vi "Perform actrion and wait for responce.vi"(7 "data step cluster":T1, 11 "error in (no error)":errorcluster) -> (2 "Rdesistance go to":bool, 3 "Voltage go to":bool, 6 "Continue":bool, 8 "Retry":bool, 13 "Stroke  go to":bool, 14 "Action value tool":dbl, 15 "error out":errorcluster)   [LabVIEW 2011]
uses:
  Sequence steps config..ctl
  Single criteria cluster.ctl
  Criteria types.ctl
  Boolean operation.ctl
  Measurments Handling/Action Analog Handler.ctl
  Measurments Handling/Common/Variable List Common Digital.ctl
  Measurments Handling/Status Digitalish.ctl
  Tool/Stroker/def/Tool specific commands.ctl
  PCP interface/High Level/PCP High Level Commands.ctl
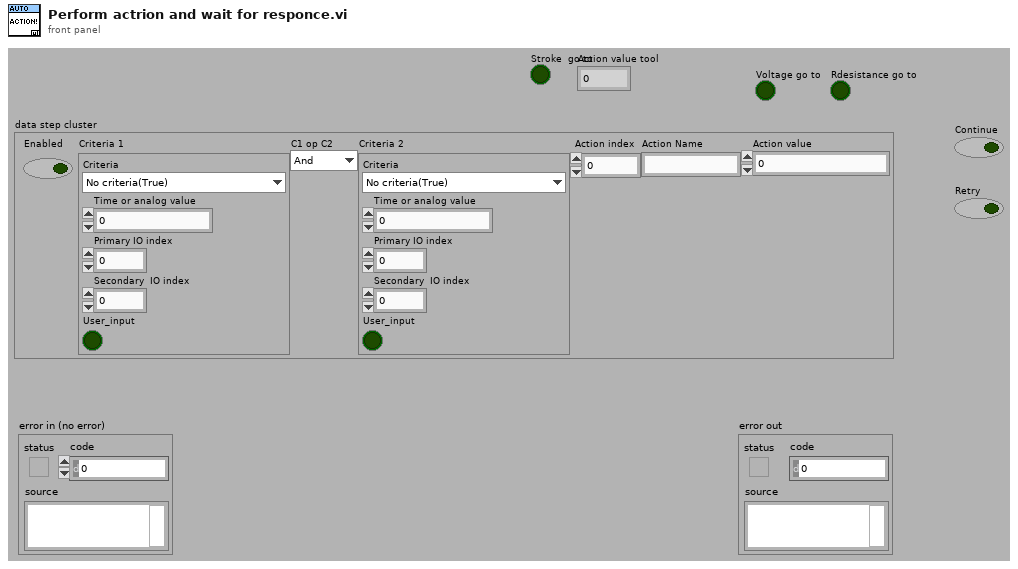
[diagram p1: front panel]
types:
  T1 = typedef "Sequence steps config..ctl" = cluster{"Enabled":bool, "Criteria 1":T2, "C1 op C2":T4, "Criteria 2":T2, "Action index":i32, "Action Name":string, "Action value":dbl}
  T2 = typedef "Single criteria cluster.ctl" = cluster{"Criteria":T3, "Time or analog value":dbl, "Primary IO index":i32, "Secondary  IO index":i32, "User_input":bool}
  T3 = typedef "Criteria types.ctl" = enum16{"No criteria(True)", "Time(s)", "Analog IO over", "Analog IO over or equal", "Analog IO under", "Analog IO under or equal", "Analog IO 1 minus Analog IO 2 over", "Digital IO True", "Digital IO False", "Operator approval"}
  T4 = typedef "Boolean operation.ctl" = enum16{"And", "Or", "Xor", "Nand", "Nor", "Nxor", "Implies"}
  T5 = typedef "PCP High Level Commands.ctl" = enum16{"HVPSU HV ON", "HVPSU HV OFF", "PCP PC", "PCP Local", "Update Motor Voltage", "Update Cable Resistance", "Final Motor Voltage", "Final Resistance"}
  T6 = typedef "Tool specific commands.ctl" = enum16{"controller relay 1 on", "controller relay 1 off", "controller relay 2 on", "controller relay 2 off", "Solonoid 1 (master) on", "Solonoid 1 (master) off", "Solonoid 2 (Stroker) on", "Solonoid 2 (Stroker) off", "Solonoid 3 (Anchor) on", "Solonoid 3 (Anchor) off", "Controller relay 1 & 2 on", "Controller relay 1 & 2 off", "Controller relay 1 on, 2 off", "Controller relay 1 off, 2 on", "STROKER tool: Stop Force Mon", "High-G Stop", "High-G Get data", "High-G Stop Get data", "STROKER tool: Stroke out", "STROKER tool: Stroke in", "STROKER tool: Stroke stop", "STROKER tool: Stroke go to", "STROKER tool: Stop Homing", "STROKER tool: Start Force Mon dir in", "STROKER tool: Start Force Mon dir out", "Controller STOP"}
  T7 = typedef "Status Digitalish.ctl" = enum16{"NA", "False", "True"}
  T8 = typedef "Variable List Common Digital.ctl" = enum16{"PCP Connected", "PCP PC Control", "HV PSU connected", "HV PSU HV Active", "Modem Connected", "Tool Connected", "CanBus interface"}
  T9 = typedef "Action Analog Handler.ctl" = enum16{"GET value", "GET Single Frequenzy", "GET All Values", "GET Waveform", "Get Numb Var", "SET Value", "START Buffer", "REG Variable", "BUF size(total antal sekund)", "PULS", "Get a Value at time", "Set initial waveform"}
  T10 = typedef "Action colleciton cluster.ctl" = cluster{"common":T11, "Action type":T13, "General command":T14, "PCP command":T5, "Tool command":T6}
  T11 = typedef "Action common elements.ctl" = cluster{"Name":string, "Adjuster type":T12, "Adjuster double default value":dbl}
  T12 = typedef "Action adjuster type.ctl" = enum16{"Non", "Double"}
  T13 = typedef "Action type.ctl" = enum16{"General", "PCP command", "Tool command"}
  T14 = typedef "General command list.ctl" = enum16{"No action"}
  T15 = enum16{"Left Button", "Center Button", "Right Button", "Window Close"}
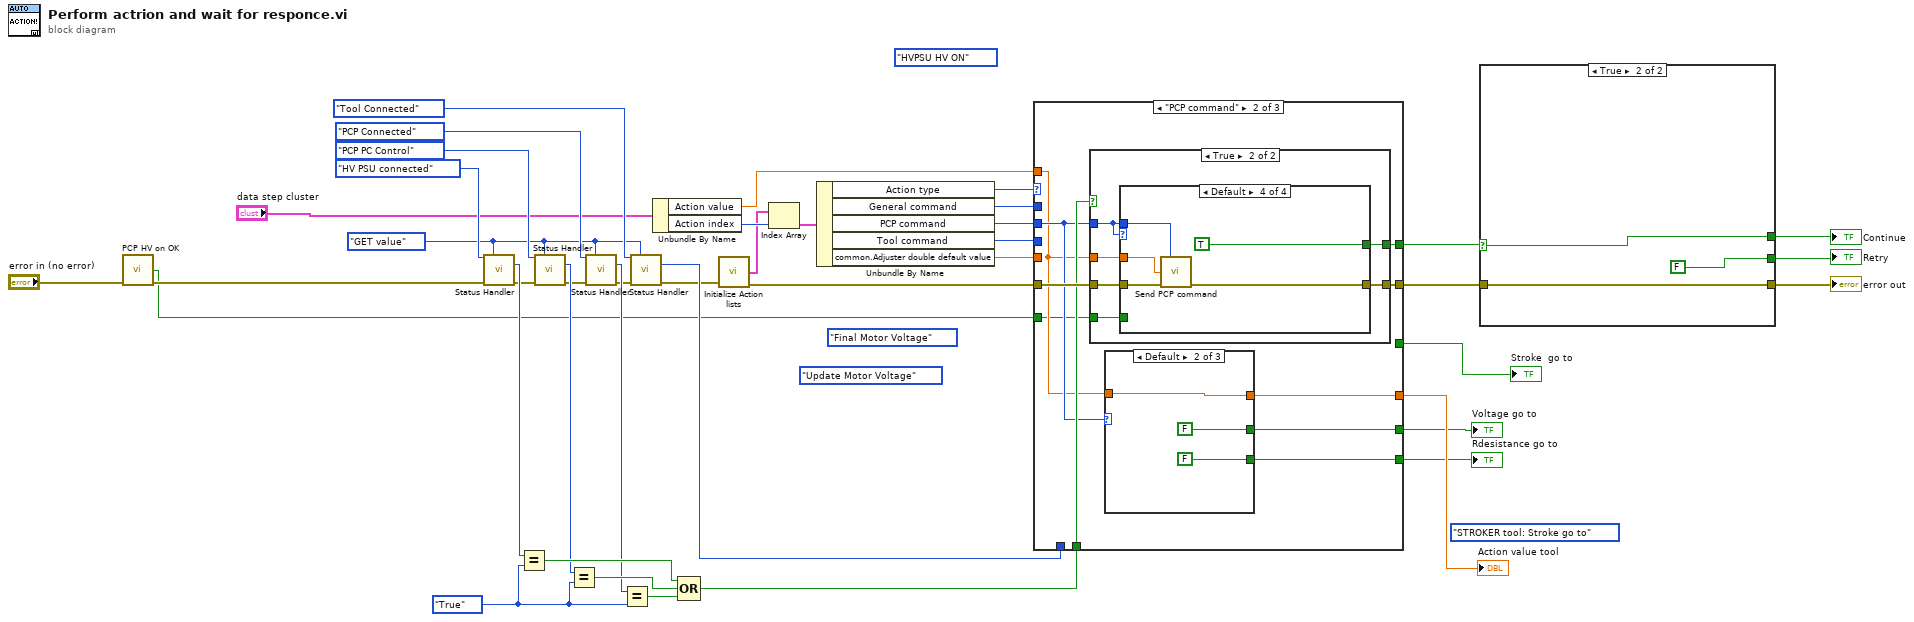
[diagram p0: block diagram]
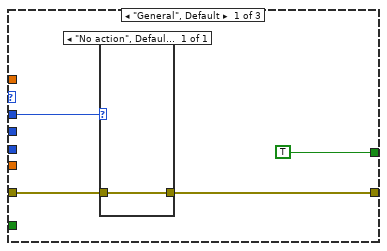
[diagram p2: hidden frame]
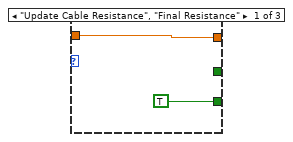
[diagram p3: hidden frame]
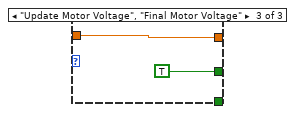
[diagram p4: hidden frame]
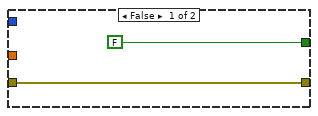
[diagram p5: hidden frame]
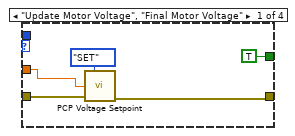
[diagram p6: hidden frame]
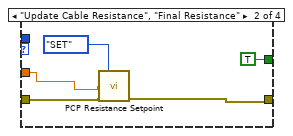
[diagram p7: hidden frame]
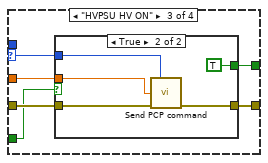
[diagram p8: hidden frame]
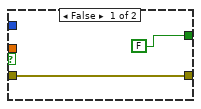
[diagram p9: hidden frame]
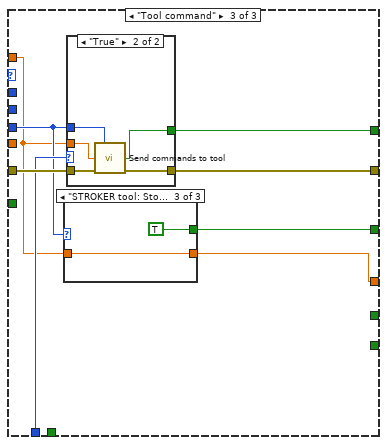
[diagram p10: hidden frame]
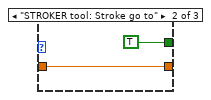
[diagram p12: hidden frame]
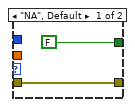
[diagram p13: hidden frame]
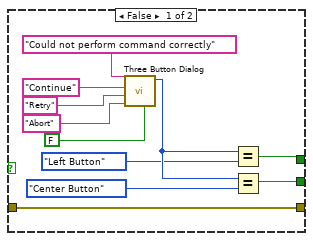
[diagram p14: hidden frame]
diagram:
  (unwired) PCP_High_Level_Commands."HVPSU HV ON" ("PCP command")
  (unwired) PCP_High_Level_Commands."Final Motor Voltage" ("PCP command")
  (unwired) PCP_High_Level_Commands."Update Motor Voltage" ("PCP command")
  (unwired) Tool_specific_commands."STROKER tool: Stroke go to" ("Tool command")
  w37 = Status_Digitalish."True" ("y")
  w9 = Action_Analog_Handler."GET value" ("Action")
  n1 = call "PCP HV on OK.vi"("error in (no error)"="error in (no error)") -> ("PCP cHV on OKout"=w1:bool, "error out"=w2:errorcluster)  [unwired: 11 in, 2 out]
  n2 = call "Status Handler.vi"("Variable Index"=Variable_List_Common_Digital."HV PSU connected" ("Action"), "Action"=w9, "error in (no error)"=w2) -> ("Value out"=w34:T7, "error out"=w32:errorcluster)  [unwired: 8 in, 3 out]
  n3 = Equal?(x=w34, y=w37) -> (x = y?=w40:bool)
  n4 = call "Status Handler.vi"("Variable Index"=Variable_List_Common_Digital."PCP PC Control" ("Action"), "Action"=w9, "error in (no error)"=w32) -> ("Value out"=w35:T7, "error out"=w25:errorcluster)  [unwired: 8 in, 3 out]
  n5 = Equal?(x=w35, y=w37) -> (x = y?=w39:bool)
  n6 = call "Status Handler.vi"("Variable Index"=Variable_List_Common_Digital."PCP Connected" ("Action"), "Action"=w9, "error in (no error)"=w25) -> ("Value out"=w36:T7, "error out"=w26:errorcluster)  [unwired: 8 in, 3 out]
  n7 = Equal?(x=w36, y=w37) -> (x = y?=w38:bool)
  n8 = call "Status Handler.vi"("Variable Index"=Variable_List_Common_Digital."Tool Connected" ("Action"), "Action"=w9, "error in (no error)"=w26) -> ("Value out"=w31:T7, "error out"=w27:errorcluster)  [unwired: 8 in, 3 out]
  n9 = Unbundle By Name("data step cluster") -> ("Action value"=w8:dbl, "Action index"=w17:i32)
  n10 = Compound Arithmetic op=OR(w40, w39, w38) -> (w41:bool)
  n11 = call "Initialize Action lists.vi"("error in (no error)"=w27) -> ("Actions"=w16:T10[], "error out"=w23:errorcluster)  [unwired: 12 in, 1 out]
  n12 = Index Array(array=w16, index=w17) -> (element=w18:T10)
  n13 = Unbundle By Name(w18) -> ("Action type"=w19:T13, "General command"=w20:T14, "PCP command"=w21:T5, "Tool command"=w22:T6, "common.Adjuster double default value"=w24:dbl)
  n14 = case shown="\"PCP command\"" w19 {
    tunnel: w20 -> [w45 _ _]
    tunnel: w21 -> [_ w52 _]
    tunnel: w22 -> [_ _ w103]
    tunnel: w23 -> [w43 w56 w107]
    tunnel: [w44 w55 w106] -> w11
    tunnel: w24 -> [_ _ _]
    tunnel: [TRUE ("Understandable reply if needed from tool") w54 w105] -> w12
    tunnel: w31 -> [_ _ w104]
    tunnel: w41 -> [_ w53 _]
    tunnel: w8 -> [_ w48 w102]
    tunnel: [_ _ w101] -> w7
    tunnel: [_ w49 w100] -> w6
    tunnel: [_ w51 _] -> w5
    tunnel: [_ w50 _] -> w4
    tunnel: w1 -> [_ w47 _]
    frame "General", Default {
      n15 = case shown="\"No action\", Default" w45 {
        tunnel: [w46] -> w44
        tunnel: w43 -> [w46]
        frame "No action", Default {
        }
      }
    }
    frame "PCP command" {
      n16 = case shown="True" w53 {
        tunnel: w56 -> [w65 w71]
        tunnel: [w65 w70] -> w55
        tunnel: w52 -> [_ w67]
        tunnel: w48 -> [_ w69]
        tunnel: [FALSE ("Understandable reply if needed from tool") w68] -> w54
        tunnel: w47 -> [_ w66]
        frame False {
        }
        frame True {
          n17 = case shown="Default" w67 {
            selector: w67 -> [_ _ w82 _]
            tunnel: w71 -> [w75 w79 w87 w99]
            tunnel: [w74 w77 w86 w98] -> w70
            tunnel: w67 -> [_ _ _ w97]
            tunnel: w69 -> [w73 w78 w83 w96]
            tunnel: [TRUE ("Understandable reply if needed from tool") TRUE ("Understandable reply if needed from tool") w84 TRUE ("Understandable reply if needed from tool")] -> w68
            tunnel: w66 -> [_ _ w85 _]
            frame "Update Motor Voltage", "Final Motor Voltage" {
              n18 = call "PCP Voltage Setpoint.vi"("Action(GET)"=enum16{"GET", "SET"}."SET", "PCP HV setpoint"=w73, "error in (no error)"=w75) -> ("error out"=w74:errorcluster)  [unwired: 11 in, 1 out]
            }
            frame "Update Cable Resistance", "Final Resistance" {
              n19 = call "PCP Resistance Setpoint.vi"("Action(GET)"=enum16{"GET", "SET"}."SET", "PCP Res setpoint"=w78, "error in (no error)"=w79) -> ("error out"=w77:errorcluster)  [unwired: 11 in, 1 out]
            }
            frame "HVPSU HV ON" {
              n20 = case shown="True" w85 {
                tunnel: w87 -> [w88 w92]
                tunnel: [w88 w91] -> w86
                tunnel: [FALSE TRUE] -> w84
                tunnel: w83 -> [_ w94]
                tunnel: w82 -> [_ w93]
                frame False {
                }
                frame True {
                  n21 = call "Send PCP command.vi"("PCP"=w93, "SP"=w94, "error out 2"=w92) -> ("error out"=w91:errorcluster)  [unwired: 9 in, 3 out]
                }
              }
            }
            frame Default {
              n22 = call "Send PCP command.vi"("PCP"=w97, "SP"=w96, "error out 2"=w99) -> ("error out"=w98:errorcluster)  [unwired: 9 in, 3 out]
            }
          }
        }
      }
      n23 = case shown="Default" w52 {
        tunnel: [_ FALSE ("Voltage go to") TRUE ("Voltage go to")] -> w51
        tunnel: [TRUE ("Rdesistance go to") FALSE ("Rdesistance go to") _] -> w50
        tunnel: [w58 w59 w63] -> w49
        tunnel: w48 -> [w58 w59 w63]
        frame "Update Cable Resistance", "Final Resistance" {
        }
        frame Default {
        }
        frame "Update Motor Voltage", "Final Motor Voltage" {
        }
      }
    }
    frame "Tool command" {
      n24 = case shown="\"STROKER tool: Stop Homing\"" w103 {
        tunnel: w102 -> [_ w108 w110]
        tunnel: [_ TRUE TRUE] -> w101
        tunnel: [_ w108 w110] -> w100
        frame Default {
        }
        frame "STROKER tool: Stroke go to" {
        }
        frame "STROKER tool: Stop Homing" {
        }
      }
      n25 = case shown="\"True\"" w104 {
        tunnel: w107 -> [w113 w118]
        tunnel: [w113 w117] -> w106
        tunnel: w103 -> [_ w116]
        tunnel: w102 -> [_ w115]
        tunnel: [FALSE ("Understandable reply if needed from tool") w114] -> w105
        frame "NA", Default {
        }
        frame "True" {
          n26 = call "Send commands to tool.vi"("Tool command"=w116, "Input Data"=w115, "error in"=w118) -> ("OK"=w114:bool, "error out"=w117:errorcluster)  [unwired: 11 in]
        }
      }
    }
  }
  "Stroke  go to" <- w7
  "Action value tool" <- w6
  "Voltage go to" <- w5
  "Rdesistance go to" <- w4
  n27 = case shown="True" w12 {
    selector: w12 -> [_ w132]
    tunnel: w11 -> [w119 w130]
    tunnel: [w124 w132] -> w13
    tunnel: [w123 FALSE] -> w14
    tunnel: [w119 w130] -> w15
    frame False {
      n28 = call <vilib>:"Three Button Dialog.vi"("Allow user to close window? (TRUE)"=FALSE, "Right Button Text (\"Cancel\")"="Abort" ("Right Button Text (\"Cancel\")"), "Center Button Text (\"No\")"="Retry" ("Center Button Text (\"No\")"), "Left Button Text (\"Yes\")"="Continue" ("Left Button Text (\"Yes\")"), "message"="Could not perform command correctly") -> ("Which Button?"=w122:T15)  [unwired: 6 in]
      n29 = Equal?(x=w122, y=T15."Left Button") -> (x = y?=w124:bool)
      n30 = Equal?(x=w122, y=T15."Center Button") -> (x = y?=w123:bool)
    }
    frame True {
    }
  }
  "error out" <- w15
  "Retry" <- w14
  "Continue" <- w13
